vi "TagToFrame(scalar)__slk_mt.vi"(8 "error in (no error)":errorcluster, 10 "tag":string, 11 "string adapter in":refnum<class "StringAdapter__slk_mt.lvclass">) -> (0 "error out":errorcluster, 2 "frame":string, 3 "string adapter out":refnum<class "StringAdapter__slk_mt.lvclass">)   [LabVIEW 2014, in "Lazyboots Menu Tool.lvlib" / "StringAdapter__slk_mt.lvclass"]
doc: "Converts tree control tag to case frame name."
uses:
  StringAdapter__slk_mt.lvclass
panel:
  # "TagToFrame(scalar)__slk_mt.vi\nConverts tree control tag to case frame name.\n\nNOTICE -- YOU MUST LEAVE THIS NOTICE IN PLACE.\n\nCopyright (c) 2011, LIANG LIU Shawn.Liu.cn@gmail.com\nAll rights reserved.\n\nRedistribution and use in source and binary forms, with or without modification, are permitted provided that the following conditions are met:\n-Redistributions of source code must retain the above copyright notice, this list of conditions and the following disclaimer.\n-Redistributions in binary form must reproduce the above copyright notice, this list of conditions and the following disclaimer in the documentation and/or other materials provided with the distribution.\n-Neither the name of the eLp nor the names of its contributors may be used to endorse or promote products derived from this software without specific prior written permission.\n\nTHIS SOFTWARE IS PROVIDED BY THE COPYRIGHT HOLDERS AND CONTRIBUTORS \"AS IS\" AND ANY EXPRESS OR IMPLIED WARRANTIES, INCLUDING, BUT NOT LIMITED TO, THE IMPLIED WARRANTIES OF MERCHANTABILITY AND FITNESS FOR A PARTICULAR PURPOSE ARE DISCLAIMED. IN NO EVENT SHALL THE COPYRIGHT HOLDER OR CONTRIBUTORS BE LIABLE FOR ANY DIRECT, INDIRECT, INCIDENTAL, SPECIAL, EXEMPLARY, OR CONSEQUENTIAL DAMAGES (INCLUDING, BUT NOT LIMITED TO, PROCUREMENT OF SUBSTITUTE GOODS OR SERVICES; LOSS OF USE, DATA, OR PROFITS; OR BUSINESS INTERRUPTION) HOWEVER CAUSED AND ON ANY THEORY OF LIABILITY, WHETHER IN CONTRACT, STRICT LIABILITY, OR TORT (INCLUDING NEGLIGENCE OR OTHERWISE) ARISING IN ANY WAY OUT OF THE USE OF THIS SOFTWARE, EVEN IF ADVISED OF THE POSSIBILITY OF SUCH DAMAGE."
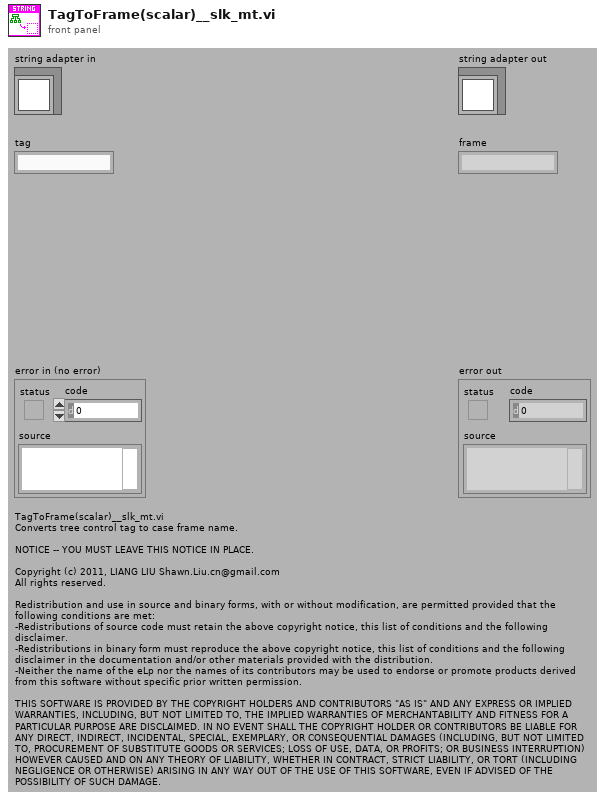
[diagram p1: front panel]
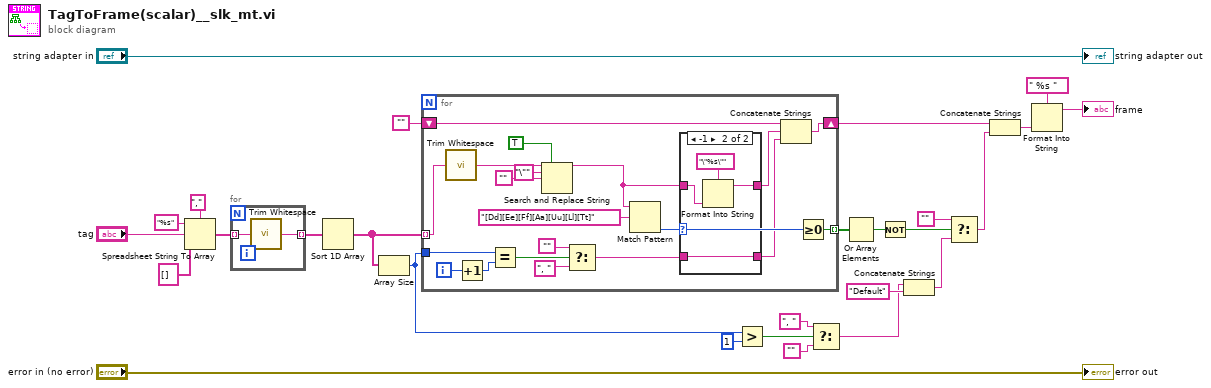
[diagram p0: block diagram]
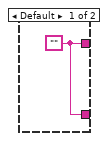
[diagram p2: hidden frame]
diagram:
  n1 = Spreadsheet String To Array(delimiter (Tab)="," ("search string"), format string="%s", spreadsheet string="tag", array type (2D Dbl)=string[] []) -> (array=w22:string[])
  n2 = for {
    tunnel: w22 -> [w29] mode=indexing
    tunnel: [w28] -> w21 mode=indexing
    n3 = call <vilib>:"Trim Whitespace.vi"("string"=w29) -> ("trimmed string"=w28:string)  [unwired: 1 in]
  }
  n4 = Sort 1D Array(array=w21) -> (sorted array=w27:string[])
  n5 = Array Size(array=w27) -> (size(s)=w12:i32)
  n6 = for {
    tunnel: w27 -> [w49] mode=indexing
    shift-right: [w48] -> w20
    shift-left: "" -> [w47]
    tunnel: w12 -> [w41]
    tunnel: [w32] -> w17 mode=indexing
    i -> [w46]
    n7 = call <vilib>:"Trim Whitespace.vi"("string"=w49) -> ("trimmed string"=w34:string)  [unwired: 1 in]
    n8 = Increment(x=w46) -> (x+1=w45:i32)
    n9 = Equal?(x=w41, y=w45) -> (x = y?=w44:bool)
    n10 = Search and Replace String(replace all?=TRUE ("replace all? (F)"), input string=w34, search string="\"", replace string="") -> (result string=w35:string)  [unwired: 4 in, 3 out]
    n11 = Select(t="", s=w44, f=", " ("search string")) -> (s? t:f=w31:string)
    n12 = Match Pattern(string=w35, regular expression="[Dd][Ee][Ff][Aa][Uu][Ll][Tt]") -> (offset past match=w33:i32)  [unwired: 1 in, 3 out]
    n13 = case shown="-1" w33 {
      tunnel: w35 -> [_ w53]
      tunnel: [w50 w52] -> w39
      tunnel: w31 -> [_ w51]
      tunnel: [w50 w51] -> w30
      frame Default {
        w50 = ""
      }
      frame -1 {
        n14 = Format Into String(format string="\"%s\"", w53) -> (resulting string=w52:string)  [unwired: 2 in, 1 out]
      }
    }
    n15 = Concatenate Strings(w47, w39, w30) -> (w48:string)
    n16 = Greater Or Equal To 0?(x=w33) -> (x >= 0?=w32:bool)
  }
  n17 = Greater?(x=w12, y=1) -> (0:w9:bool)
  n18 = Select(t=", " ("x"), s=w9, f="") -> (s? t:f=w7:string)
  n19 = Or Array Elements(Boolean array=w17) -> (logical OR=w16:bool)
  n20 = Not(x=w16) -> (.not. x?=w14:bool)
  n21 = Concatenate Strings(w7, "Default" ("x")) -> (w5:string)
  n22 = Select(t="", s=w14, f=w5) -> (s? t:f=w15:string)
  n23 = Concatenate Strings(w20, w15) -> (w18:string)
  n24 = Format Into String(format string=" %s ", w18) -> (resulting string=→"frame":string)  [unwired: 2 in, 1 out]
  "error out" <- "error in (no error)"
  "string adapter out" <- "string adapter in"
